vi "Single Calculation.vi"(1 "Array Input":dbl[](array[numeric])) -> (0 "Array Output":dbl[](array[numeric]))   [LabVIEW 2020]
panel:
  out "Charging Voltage":dbl
  out "Total\nTemperature Change":dbl
  out "Energy Loss":dbl
  out "Power Loss":dbl
  out "Charging Time":dbl
  out "Charing Current":dbl
  out "J in 1 NS pair with gap":dbl
  out "Energy (wh/m3) / 1 NS pari with gap":dbl
  out "Energy Density  WH/m3":dbl
  out "Energy Density  WH/Lit":dbl
  out "1 NS Pair Energy / Volume":dbl
  out "1 NS Pair Energy / mass":dbl
  out "Chip Energy Wh":dbl
  out "WH/Lit":dbl
  out "WH/m3":dbl
  out "WH/Kg":dbl
  out "Chip Energy / Volume":dbl
  out "Chip Energy /Mass":dbl
  out "Mass of a Chip":dbl
  out "Volume of a Chip":dbl
  out "Mass NS Pair with Gap":dbl
  out "Volume NS Pair With Gap":dbl
  out "Volume Gap":dbl
  out "Mass Gap":dbl
  out "Delta Temp Change \nDielectric Gap":dbl
  out "Dielectric Thickness  \nGap":dbl
  out "Mass Dielectric \nGap":dbl
  out "Volume Dielectric \nGap":dbl
  out "Delta Temp Change\n SiO2 Gap":dbl
  out "Mass SiO2 Gap":dbl
  out "Sio2 Thickness Gap":dbl
  out "Volume SiO2 Gap":dbl
  out "Volume Si Gap":dbl
  out "Silicon Thickness Gap":dbl
  out "Mass Si Gap":dbl
  out "Delta Temp Change\n Si Gap":dbl
  out "Area B/W NS":dbl
  out "Vol 2 NS":dbl
  out "Mass 2 NS":dbl
  out "Mass 1 NS":dbl
  out "Volume 1 NS":dbl
  out "SiO2 Specfic Heat Capacity 2":dbl
  out "SilO2 Density 2":dbl
  out "Delta Temp Change SiO2 2":dbl
  out "Mass SiO2 2":dbl
  out "Volume SiO2 2":dbl
  out "Dielectric Specfic Heat Capacity":dbl
  out "Dielectric Density":dbl
  out "CNT Specfic Heat Capacity":dbl
  out "CNT Density":dbl
  out "Fe Specfic Heat Capacity":dbl
  out "Fe Density":dbl
  out "Al Specfic Heat Capacity":dbl
  out "Al Density":dbl
  out "Al2O3 Specfic Heat Capacity":dbl
  out "Al2O3 Density":dbl
  out "M1 Specfic Heat Capacity":dbl
  out "M1 Density":dbl
  out "SiO2 Specfic Heat Capacity":dbl
  out "SilO2 Density":dbl
  out "um in 1 inch":dbl
  out "Microns":dbl
  out "Inches":dbl
  out "Energy (Heat; I^2R)":dbl
  out "Delta Temp Change \nDielectric":dbl
  out "Mass Dielectric":dbl
  out "Volume Dielectric":dbl
  out "Delta Temp Change CNT":dbl
  out "Mass CNTs":dbl
  out "Volume CNT":dbl
  out "Delta Temp Change Fe":dbl
  out "Mass Fe":dbl
  out "Volume Fe":dbl
  out "Delta Temp Change Al":dbl
  out "Mass  Al":dbl
  out "Volume Al":dbl
  out "Delta Temp Change Al2O3":dbl
  out "Mass Al2O3":dbl
  out "Volume Al2O3":dbl
  out "Delta Temp Change M1":dbl
  out "Mass M1":dbl
  out "Volume M1":dbl
  out "Delta Temp Change SiO2":dbl
  out "Mass SiO2":dbl
  out "Volume SiO2":dbl
  out "Dielectric Thickness":dbl
  out "CNT Thickness":dbl
  out "Fe Thickness":dbl
  out "Al Thickness":dbl
  out "Al2O3 Thickness":dbl
  out "M1 Thickness":dbl
  out "SiO2 Thickness 2":dbl
  out "Sio2 Thickness":dbl
  out "Silicon Thickness":dbl
  out "m-nm Dielectric":dbl
  out "Dielectric Thickness":dbl
  out "m-nm CNT":dbl
  out "CNT Thickness (CNT Length)":dbl
  out "m-nm Fe":dbl
  out "Fe Thickness":dbl
  out "m-nm Al":dbl
  out "Aluminum Thickness":dbl
  out "Heat Generated (Energy) by Current in Metal films":dbl
  out "Delta Temp Change Si":dbl
  out "Silicon Specfic Heat Capacity":dbl
  out "Silicon Density":dbl
  out "Mass Si":dbl
  out "Volume Si":dbl
  out "m-nm SiO2 2":dbl
  out "Silicon DiOxide Thickness  2":dbl
  out "m-nm Al2O3":dbl
  out "m-nm M1":dbl
  out "Alumina Thickness":dbl
  out "Metal 1 (Ti)":dbl
  out "m-nm SiO2":dbl
  out "m-nm Si":dbl
  out "Silicon DiOxide Thickness":dbl
  out "Silicon Thickness":dbl
  out "Rf for Max i;  R+ C (EDL+Funct)":dbl
  out "Rf for Max i;  R+ C (EDL+Funct+ Analyte)":dbl
  out "Max V_out":dbl
  out "Delta i":dbl
  out "Max i;  R+ C (EDL+Funct+ Analyte)":dbl format="%#_9e"
  out "Max i;  R+ C (EDL+Funct)":dbl format="%#_9e"
  out "V_Zeta":dbl
  out "|Z| of R+ C (EDL+Funct+Analyte)":dbl
  out "|Z| of R+ C (EDL+Funct)":dbl
  out "Delta Total Impedance":dbl
  out "Total Impedance Rs+C(EDS+Funct+Analyte)":dbl
  out "Total Impedance Rs+C(EDS+Funct)":dbl
  out "Series Resistance of Solution":dbl
  out "Freq Hz-MHz":dbl
  out "Impedance of EDL & Functionalization & Analyte":dbl
  out "Impedance of EDL & Functionalization":dbl
  out "Frequency":dbl
  out "Delta C":dbl
  out "Capacitance of ELD & Functionalization & Analyte":dbl
  out "Capacitance of ELD & Functionalization":dbl
  out "C_EDL/ 1 NS":dbl
  out "C_EDL/ 1 CNT":dbl
  out "C EDL by d with Cosh Factor":dbl format="%#_6e"
  out "C EDL by d":dbl
  out "d; EDL Length":dbl
  out "R=kN_a":dbl
  out "F=eN_a":dbl
  out "N_a; Avagadro no":dbl=1.38064852e-23
  out "V  nV-m V-V":dbl
  out "C_EDL/ A":dbl format="%#_6e"
  out "c; Charge on e":dbl=1.6021766208e-19
  out "V zeta":dbl
  out "C in M":dbl
  out "Co nM-M":dbl
  out "T":dbl
  out "k; Boltzmann Constant":dbl=1.38064852e-23
  out "Co; miliMolar (moles/m3)":dbl
  out "er":dbl
  out "eo; Permitivity of Free Space":dbl=8.85418782e-12
  out "z":dbl
  out "Length of CNTs  2":dbl
  out "Dielectric of Molecule 2 Analyte":dbl
  out "Capacitance Functinal Analyte  per unit area":dbl
  out "Capaciatance per CNT Analyte":dbl
  out "Capacitance Functional Analyte per NS":dbl
  out "Capacitance Functional Analyte per NS 2":dbl
  out "Gap B/w NS":dbl
  out "Chip Impedance":dbl
  out "Chip Capacitance":dbl
  out "Chip Energy":dbl
  out "Chip Power":dbl
  out "Freq Hz K; M Hz":dbl
  out "Power":dbl
  out "Frequency":dbl
  out "Impedance":dbl
  out "Voltage":dbl
  out "Energy":dbl
  out "Capacitance of 1 Pair NS":dbl(graph)
  out "Capacitance of 1 Pair NS":dbl
  out "er":dbl
  out "Capacitance Functional Molecules per NS 2":dbl
  out "Capacitance Functional Molecules per NS":dbl
  out "Capaciatance per CNT Functional":dbl
  out "Capacitance Functinal Molecule  per unit area":dbl
  out "Dielectric of Molecule":dbl
  out "Concentration,  M":dbl[unit]
  out "Concentration on 1 NS (Moles/m3)":dbl[unit]
  out "Total Functionalized Molecules on NS":dbl
  out "No of Molecules on 1 CNT Functionalized":dbl
  out "Molecule Length Analyte":dbl
  out "Molecle Area with Gap Analyte":dbl
  out "Volume of Molecule Analyte":dbl
  out "Area of Molecule on CNT surface Analyte":dbl
  out "m-nm Gap Molecules Analyte":dbl caption="m-nm Gap"
  out "Gap Between Molecules Analyte":dbl caption="Gap Between CNTs"
  out "m-nm l Molecule Analyte":dbl
  out "m-nm r Molecule Analyte":dbl caption="m-nm r"
  out "Length of Molecule Analyte":dbl caption="Length of CNTs"
  out "Radius of Molecule Analyte":dbl caption="Radius of CNTs"
  out "Molecule Length":dbl
  out "Molecle Area with Gap":dbl
  out "Volume of Molecule":dbl
  out "Area of Molecule on CNT surface":dbl
  out "m-nm Gap Molecules":dbl caption="m-nm Gap"
  out "Gap Between Molecules":dbl caption="Gap Between CNTs"
  out "m-nm l Molecule":dbl
  out "m-nm r Molecule":dbl caption="m-nm r"
  out "Length of Molecule":dbl caption="Length of CNTs"
  out "Radius of Molecule":dbl caption="Radius of CNTs"
  out "NS Width":dbl
  out "No of NS Pairs on Chip":dbl
  out "Gap n-m":dbl
  out "Gap B/W NS":dbl
  out "m-nm LChip":dbl
  out "m-nm WChip":dbl
  out "Length of Chip":dbl
  out "Width of Chip":dbl
  out "Surface Area 1 NS":dbl
  out "# of CNTs in 1 NS":dbl format="%#_6e"
  out "Area 1 CNT & Gap":dbl
  out "NS Length":dbl
  out "NS Base Area":dbl
  out "CNT Radius":dbl
  out "CNT Base Area":dbl
  out "XY Graph":cluster{"X":dbl[], "Y":dbl[]}[](graph)
  out "m-nm NS Base":dbl caption="m-nm 4"
  out "m-nm WB":dbl
  out "Length of Base":dbl
  out "Width of Base":dbl
  out "m-nm Gap":dbl
  out "Gap Between CNTs":dbl
  out "Surface Area of 1 CNT":dbl
  out "m-nm l":dbl
  out "m-nm r":dbl
  out "Length of CNTs":dbl
  out "Radius of CNTs":dbl
  # "CAP"
  # "Chip CAP"
  # "Chip NanoStructure"
  # "CNT Nanostructure"
  # "CAP Design"
  # "Nano Structure Material Stack"
  # "Constants for Materials in Stack"
  # "Nano Structure"
  # "Charging/Discharging"
  # "Chip"
  # "Dielectric =1/2 of Gap B/w NS"
  # "Analyte Molecule"
  # "Functionalization Molecule"
  # "Analyte Attached to Functionalized  NanoStructure"
  # "TiO2: 4260 kg/m3\nHafnium Odide: 9680"
  # "GAP B/W NS  Material"
  # "Capacitance of Analyte Molecule on NanoStructure"
  # "Functionalized NanoStructure"
  # "Mass and Volume of NS Pair"
  # "Molecule Fnctionalization"
  # "Capacitance of Functional Molecule on NanoStructure"
  # "Mass and Volume of Chip"
  # "Echem & Electrical Signals"
  # "Electric Double Layer; EDL"
  # "Constants"
  # "Cosh(zeV_zeta/2kT)"
  # "Potentiostat"
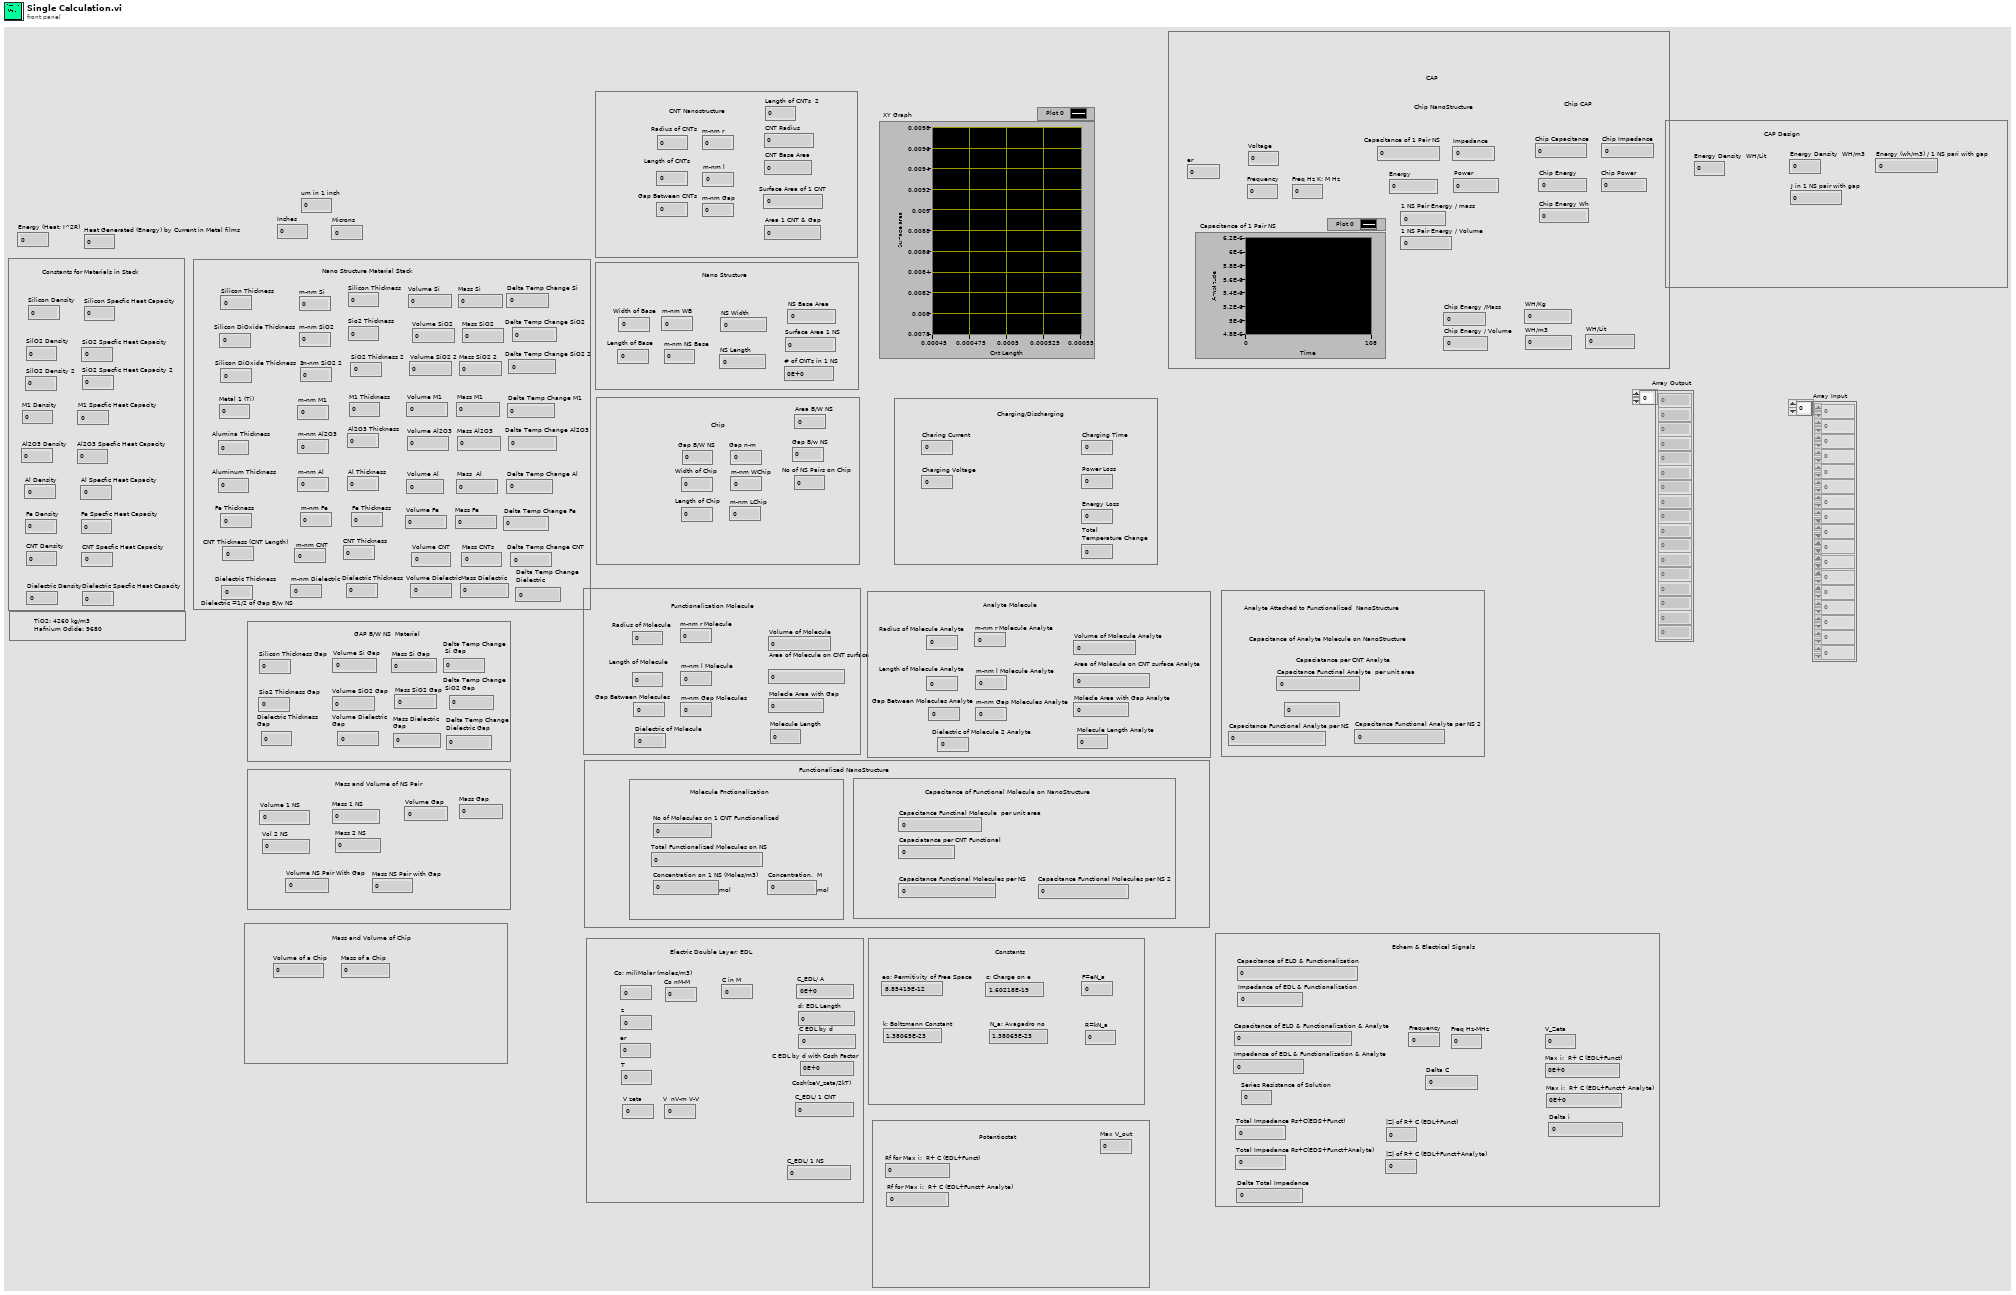
[diagram p1: front panel]
types:
  T1 = cluster{"Array Input[0]":dbl, "Array Input[1]":dbl, "Array Input[2]":dbl, "Array Input[3]":dbl, "Array Input[4]":dbl, "Array Input[5]":dbl, "Array Input[6]":dbl, "Array Input[7]":dbl, "Array Input[8]":dbl, "Array Input[9]":dbl, "Array Input[10]":dbl, "Array Input[11]":dbl, "Array Input[12]":dbl, "Array Input[13]":dbl, "Array Input[14]":dbl, "Array Input[15]":dbl, "Array Input[16]":dbl, "Array Input[17]":dbl, "Array Input[18]":dbl, "Array Input[19]":dbl, "Array Input[20]":dbl, "Array Input[21]":dbl, "Array Input[22]":dbl, "Array Input[23]":dbl, "Array Input[24]":dbl, "Array Input[25]":dbl, "Array Input[26]":dbl, "Array Input[27]":dbl, "Array Input[28]":dbl, "Array Input[29]":dbl, "Array Input[30]":dbl, "Array Input[31]":dbl, "Array Input[32]":dbl, "Array Input[33]":dbl, "Array Input[34]":dbl, "Array Input[35]":dbl, "Array Input[36]":dbl, "Array Input[37]":dbl, "Array Input[38]":dbl, "Array Input[39]":dbl, "Array Input[40]":dbl, "Array Input[41]":dbl, "Array Input[42]":dbl, "Array Input[43]":dbl, "Array Input[44]":dbl, "Array Input[45]":dbl, "Array Input[46]":dbl, "Array Input[47]":dbl, "Array Input[48]":dbl, "Array Input[49]":dbl, "Array Input[50]":dbl, "Array Input[51]":dbl, "Array Input[52]":dbl, "Array Input[53]":dbl, "Array Input[54]":dbl, "Array Input[55]":dbl, "Array Input[56]":dbl, "Array Input[57]":dbl, "Array Input[58]":dbl, "Array Input[59]":dbl, "Array Input[60]":dbl, "Array Input[61]":dbl, "Array Input[62]":dbl, "Array Input[63]":dbl}
  T2 = cluster{"Capacitance of 1 Pair NS":dbl, "Energy":dbl, dbl, dbl, "Impedance":dbl, "Power":dbl, dbl, dbl, "Chip Capacitance":dbl, "Chip Energy":dbl, dbl, dbl, dbl, "Chip Impedance":dbl, "Chip Power":dbl, dbl, dbl, dbl, dbl, "Volume of Molecule":dbl, "Area of Molecule on CNT surface":dbl, "Molecle Area with Gap":dbl, "Molecule Length":dbl, "Capacitance Functinal Analyte  per unit area":dbl, "Capaciatance per CNT":dbl, "Capacitance Functional Analyte per NS 2":dbl, "Capacitance Functional Analyte per NS 2":dbl, "Volume of Molecule":dbl, "Area of Molecule on CNT surface":dbl, "Molecle Area with Gap":dbl, "Molecule Length":dbl, "No of Molecules on 1 CNT Functionalized ":dbl, "Total Functionalized Molecules on NS":dbl, dbl, dbl, "Capacitance Functinal Molecule  per unit area":dbl, "Capaciatance per CNT":dbl, "Capacitance Functional Molecules per NS":dbl, "Capacitance Functional Molecules per NS 2":dbl, "eo; Permitivity of Free Space":dbl, "c; Charge on e":dbl, "F=eN_a":dbl, "k; Boltzmann Constant":dbl, "N_a; Avagadro no":dbl, "R=kN_a":dbl, "C in M":dbl, "C_EDL/ A":dbl, "d; EDL Length":dbl, "C EDL by d":dbl, "C EDL by d with Cosh Factor":dbl, "C_EDL/ 1 CNT":dbl, "C_EDL/ 1 NS":dbl, dbl, dbl, "Capacitance of ELD & Functionalization":dbl, "Impedance of EDL & Functionalization":dbl, "Capacitance of ELD & Functionalization & Analyte":dbl, "Impedance of EDL & Functionalization & Analyte":dbl, "Total Impedance Rs+C(EDS+Funct)":dbl, "Total Impedance Rs+C(EDS+Funct+Analyte)":dbl, "Delta Total Impedance":dbl, "Delta C":dbl, "|Z| of R+ C (EDL+Funct)":dbl, "|Z| of R+ C (EDL+Funct+Analyte)":dbl, "V_Zeta out":dbl, "Max i;  R+ C (EDL+Funct) ":dbl, "Max i;  R+ C (EDL+Funct+ Analyte) ":dbl, "Delta i":dbl, dbl, dbl, dbl, dbl, dbl, dbl, dbl, dbl, dbl, dbl, "Silicon Thickness out":dbl, "Sio2 Thickness":dbl, "Dielectric Thickness  out":dbl, "Volume Si":dbl, "Volume SiO2":dbl, "Volume Dielectric":dbl, "Mass Si":dbl, "Mass SiO2":dbl, "Mass Dielectric":dbl, "Delta Temp Change Si":dbl, "Delta Temp Change SiO2":dbl, "Delta Temp Change \nDielectric":dbl, "Array Input[1]":dbl, dbl, "Array Input[4]":dbl, "Array Input[29]":dbl, "Silicon Thickness out":dbl, "Sio2 Thickness":dbl, "SiO2 Thickness 2":dbl, "M1 Thickness":dbl, "Al2O3 Thickness":dbl, "Al Thickness":dbl, "Fe Thickness 2":dbl, "CNT Thickness":dbl, "Dielectric Thickness  out":dbl, "Volume Si":dbl, "Volume SiO2":dbl, "Volume SiO2 2":dbl, "Volume M1":dbl, "Volume Al2O3":dbl, "Volume Al":dbl, "Volume Fe":dbl, "Volume CNT":dbl, "Volume Dielectric":dbl, "Mass Si":dbl, "Mass SiO2":dbl, "Mass SiO2 2":dbl, "Mass M1":dbl, "Mass Al2O3":dbl, "Mass  Al":dbl, "Mass Fe":dbl, "Mass CNTs":dbl, "Mass Dielectric":dbl, "Delta Temp Change Si":dbl, "Delta Temp Change SiO2":dbl, "Delta Temp Change SiO2 2":dbl, "Delta Temp Change M1":dbl, "Delta Temp Change Al2O3":dbl, "Delta Temp Change Al":dbl, "Delta Temp Change Fe":dbl, "Delta Temp Change CNT":dbl, "Delta Temp Change \nDielectric":dbl, dbl, "y":dbl, dbl, dbl, "Gap B/w NS":dbl, "No of NS Pairs on Chip":dbl, "NS Width":dbl, "NS Length":dbl, "NS Base Area":dbl, "Surface Area 1 NS":dbl, "# of CNTs in 1 NS":dbl, "Length of CNTs ":dbl, "CNT Radius":dbl, "CNT Base Area":dbl, "Surface Area of 1 CNT":dbl, "Area 1 CNT & Gap":dbl, "Silicon Density":dbl, "SilO2 Density":dbl, "SilO2 Density 2":dbl, "M1 Density":dbl, "Al2O3 Density":dbl, "Al Density":dbl, "Fe Density":dbl, "CNT Density":dbl, "Dielectric Density":dbl, "Silicon Specfic Heat Capacity":dbl, "SiO2 Specfic Heat Capacity":dbl, "SiO2 Specfic Heat Capacity 2":dbl, "M1 Specfic Heat Capacity":dbl, "Al2O3 Specfic Heat Capacity":dbl, "Al Specfic Heat Capacity":dbl, "Fe Specfic Heat Capacity":dbl, "CNT Specfic Heat Capacity":dbl, "Dielectric Specfic Heat Capacity":dbl, dbl, dbl, dbl, dbl}
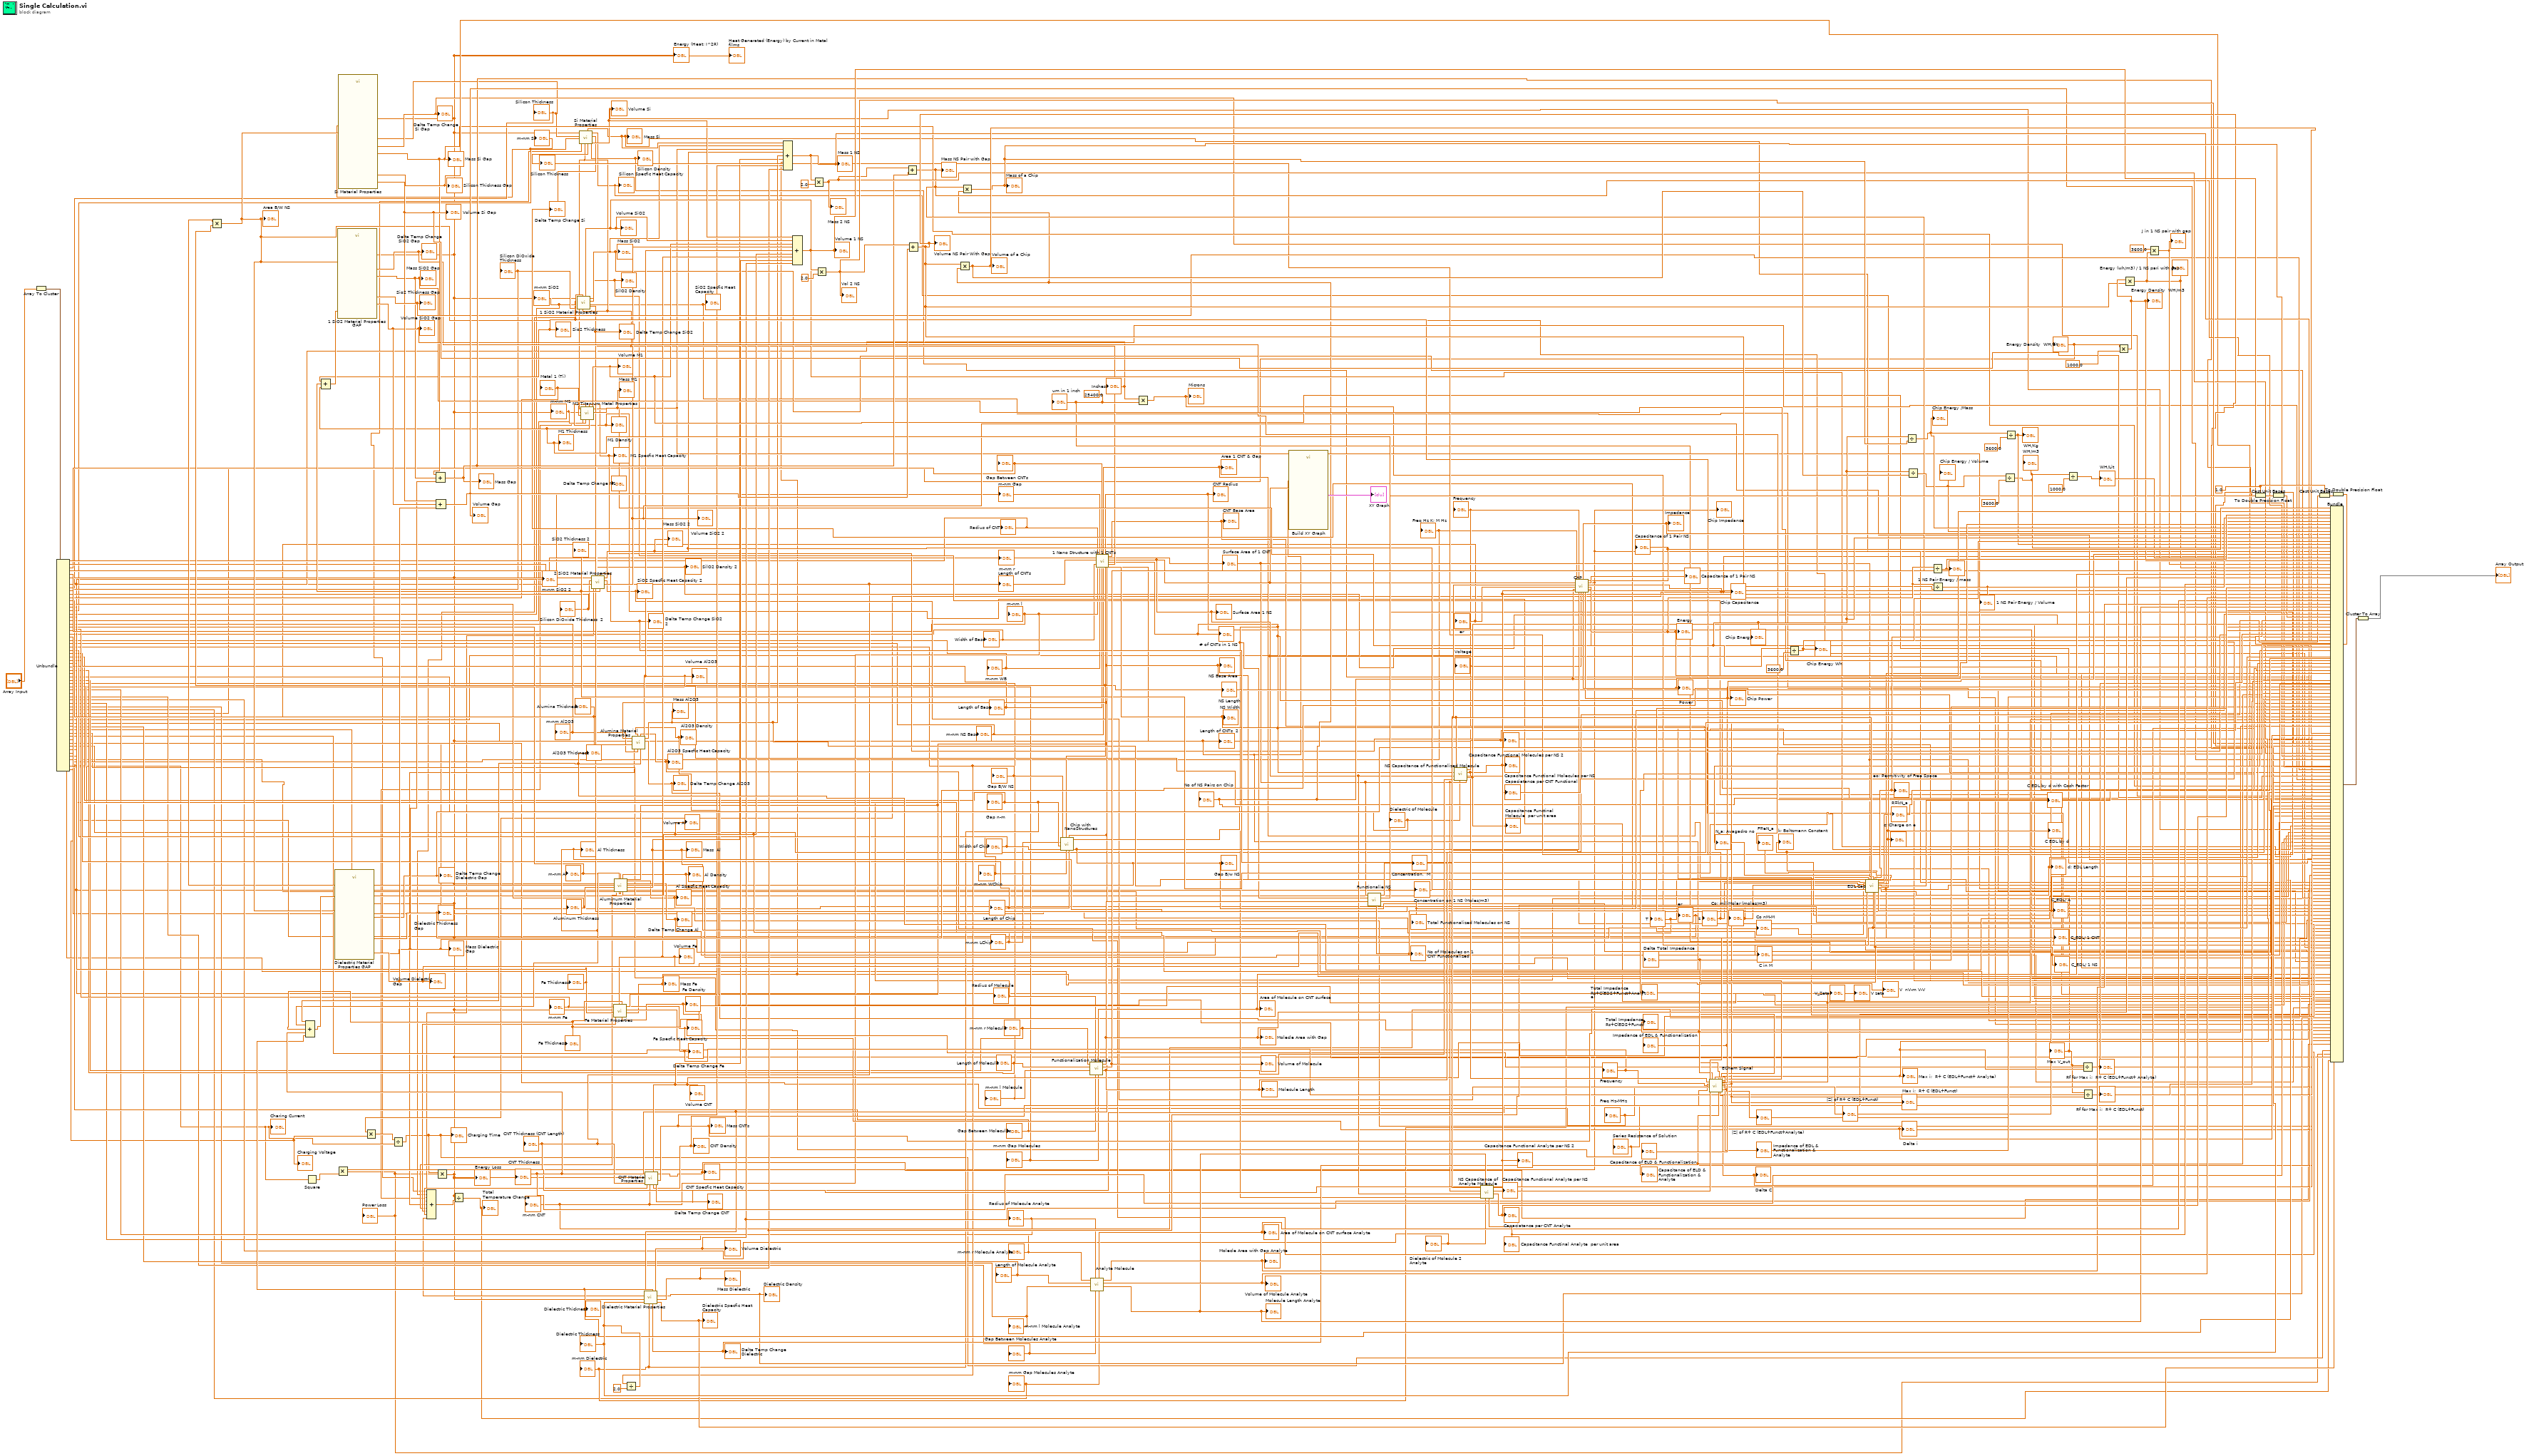
[diagram p0: block diagram]
diagram:
  w205 = 1.0
  w116 = 25400.0 ("y")
  n1 = Array To Cluster(array="Array Input") -> (cluster=w246:T1)
  n2 = Unbundle(w246) -> ("Array Input[0]"=w82:dbl, "Array Input[1]"=w81:dbl, "Array Input[2]"=w80:dbl, "Array Input[3]"=w79:dbl, "Array Input[4]"=w78:dbl, "Array Input[5]"=w77:dbl, "Array Input[7]"=w76:dbl, "Array Input[8]"=w75:dbl, "Array Input[9]"=w74:dbl, "Array Input[10]"=w73:dbl, "Array Input[11]"=w72:dbl, "Array Input[12]"=w71:dbl, "Array Input[13]"=w70:dbl, "Array Input[14]"=w69:dbl, "Array Input[15]"=w68:dbl, "Array Input[16]"=w67:dbl, "Array Input[17]"=w66:dbl, "Array Input[18]"=w65:dbl, "Array Input[19]"=w64:dbl, "Array Input[20]"=w63:dbl, "Array Input[21]"=w62:dbl, "Array Input[22]"=w61:dbl, "Array Input[23]"=w60:dbl, "Array Input[24]"=w59:dbl, "Array Input[25]"=w58:dbl, "Array Input[26]"=w57:dbl, "Array Input[27]"=w56:dbl, "Array Input[28]"=w55:dbl, "Array Input[29]"=w54:dbl, "Array Input[30]"=w53:dbl, "Array Input[31]"=w52:dbl, "Array Input[32]"=w51:dbl, "Array Input[33]"=w50:dbl, "Array Input[34]"=w49:dbl, "Array Input[35]"=w48:dbl, "Array Input[36]"=w47:dbl, "Array Input[37]"=w46:dbl, "Array Input[38]"=w45:dbl, "Array Input[39]"=w44:dbl, "Array Input[40]"=w43:dbl, "Array Input[41]"=w42:dbl, "Array Input[42]"=w41:dbl, "Array Input[43]"=w40:dbl, "Array Input[44]"=w39:dbl, "Array Input[45]"=w38:dbl, "Array Input[46]"=w37:dbl, "Array Input[47]"=w36:dbl, "Array Input[48]"=w35:dbl, "Array Input[49]"=w34:dbl, "Array Input[50]"=w33:dbl, "Array Input[51]"=w32:dbl, "Array Input[52]"=w31:dbl, "Array Input[53]"=w30:dbl, "Array Input[54]"=w29:dbl, "Array Input[55]"=w28:dbl, "Array Input[56]"=w27:dbl, "Array Input[57]"=w26:dbl, "Array Input[58]"=w25:dbl, "Array Input[59]"=w24:dbl, "Array Input[60]"=w23:dbl, "Array Input[61]"=→"V  nV-m V-V":dbl, "Array Input[62]"=w17:dbl, "Array Input[63]"=w19:dbl)  [unwired: 1 out]
  "Radius of CNTs" <- w82
  "Length of CNTs" <- w81
  "m-nm r" <- w79
  "m-nm l" <- w78
  "Gap Between CNTs" <- w80
  "m-nm Gap" <- w77
  "Width of Base" <- w61
  "Length of Base" <- w60
  "m-nm WB" <- w59
  "m-nm NS Base" <- w58
  "Width of Chip" <- w56
  "Length of Chip" <- w55
  "m-nm WChip" <- w53
  "m-nm LChip" <- w52
  "Gap B/W NS" <- w57
  "Gap n-m" <- w54
  "Radius of Molecule" <- w51
  "Length of Molecule" <- w50
  "m-nm r Molecule" <- w47
  "m-nm l Molecule" <- w46
  "Gap Between Molecules" <- w49
  "m-nm Gap Molecules" <- w45
  "Radius of Molecule Analyte" <- w44
  "Length of Molecule Analyte" <- w43
  "m-nm r Molecule Analyte" <- w40
  "m-nm l Molecule Analyte" <- w39
  "Gap Between Molecules Analyte" <- w42
  "m-nm Gap Molecules Analyte" <- w38
  "Dielectric of Molecule" <- w48
  "er" <- w36
  "Voltage" <- w35
  "Frequency" <- w34
  "Freq Hz K; M Hz" <- w33
  "Dielectric of Molecule 2 Analyte" <- w41
  "z" <- w27
  "er" <- w26
  "Co; miliMolar (moles/m3)" <- w28
  "T" <- w25
  "Co nM-M" <- w23
  "V zeta" <- w24
  "Frequency" <- w30
  "Freq Hz-MHz" <- w29
  "Series Resistance of Solution" <- w31
  "Max V_out" <- w32
  "Silicon Thickness" <- w75
  "Silicon DiOxide Thickness" <- w74
  "m-nm Si" <- w68
  "m-nm SiO2" <- w67
  "Metal 1 (Ti)" <- w72
  "Alumina Thickness" <- w71
  "m-nm M1" <- w65
  "m-nm Al2O3" <- w64
  "Silicon DiOxide Thickness  2" <- w73
  "m-nm SiO2 2" <- w66
  "Aluminum Thickness" <- w70
  "m-nm Al" <- w63
  "Fe Thickness" <- w69
  "m-nm Fe" <- w62
  "CNT Thickness (CNT Length)" <- w81
  "m-nm CNT" <- w78
  "m-nm Dielectric" <- w54
  "Inches" <- w76
  "Energy Density  WH/Lit" <- w37
  "Charing Current" <- w17
  "Charging Voltage" <- w19
  n3 = Square(x=w17) -> (x^2=w16:dbl)
  n4 = Divide(x=w57, y=2.0) -> (x/y=w152:dbl)
  "Dielectric Thickness" <- w152
  n5 = call "Functionalization Molecule.vi"("m-nm Gap Molecules"=w45, "Gap Between Molecules"=w49, "Radius of Molecule"=w51, "m-nm l Molecule"=w46, "Length of Molecule"=w50, "m-nm r Molecule"=w47) -> ("Molecule Length"=w225:dbl, "Volume of Molecule"=w228:dbl, "Molecle Area with Gap"=w226:dbl, "Area of Molecule on CNT surface"=w227:dbl)  [unwired: 2 in]
  "Area of Molecule on CNT surface" <- w227
  "Volume of Molecule" <- w228
  "Molecle Area with Gap" <- w226
  "Molecule Length" <- w225
  n6 = call "Analyte Molecule.vi"("m-nm Gap Molecules"=w38, "Gap Between Molecules"=w42, "Radius of Molecule"=w44, "m-nm l Molecule"=w39, "Length of Molecule"=w43, "m-nm r Molecule"=w40) -> ("Molecule Length"=w218:dbl, "Volume of Molecule"=w221:dbl, "Molecle Area with Gap"=w219:dbl, "Area of Molecule on CNT surface"=w220:dbl)  [unwired: 2 in]
  "Area of Molecule on CNT surface Analyte" <- w220
  "Volume of Molecule Analyte" <- w221
  "Molecle Area with Gap Analyte" <- w219
  "Molecule Length Analyte" <- w218
  n7 = call "1 Nano Structure with 1 CNTs.vi"("Radius of CNTs"=w82, "m-nm r"=w79, "Length of CNTs"=w81, "m-nm l"=w78, "Width of Base"=w61, "m-nm Gap"=w77, "m-nm WB"=w59, "Gap Between CNTs"=w80, "Length of Base"=w60, "m-nm NS Base"=w58) -> ("Length of CNTs"=w106:dbl, "Area 1 CNT & Gap"=w102:dbl, "CNT Radius"=w105:dbl, "NS Length"=w110:dbl, "CNT Base Area"=w104:dbl, "Surface Area of 1 CNT"=w103:dbl, "Surface Area 1 NS"=w108:dbl, "# of CNTs in 1 NS"=w107:dbl, "NS Base Area"=w109:dbl, "NS Width"=w111:dbl)
  "Surface Area of 1 CNT" <- w103
  "CNT Base Area" <- w104
  "CNT Radius" <- w105
  "NS Base Area" <- w109
  "NS Length" <- w110
  "Area 1 CNT & Gap" <- w102
  "# of CNTs in 1 NS" <- w107
  "Surface Area 1 NS" <- w108
  "NS Width" <- w111
  "Length of CNTs  2" <- w106
  n8 = call "Chip with NanoStructures.vi"("Length of Chip"=w55, "NS Base Area"=w109, "m-nm WChip"=w53, "NS Length"=w110, "Width of Chip"=w56, "Gap n-m"=w54, "m-nm LChip"=w52, "Gap B/W NS"=w57) -> ("Gap B/w NS"=w113:dbl, "No of NS Pairs on Chip"=w112:dbl)  [unwired: 2 in]
  "No of NS Pairs on Chip" <- w112
  "Gap B/w NS" <- w113
  n9 = Multiply(x=w113, y=w110) -> (x*y=w114:dbl)
  "Area B/W NS" <- w114
  n10 = Multiply(x=w76, y=w116) -> (x*y=w115:dbl)
  "Microns" <- w115
  n11 = call "Build XY Graph"("Y Input"=w108, "X Input"=w106) -> ("XY Graph"=→"XY Graph":cluster{"X":dbl[], "Y":dbl[]}[])  [unwired: 8 in, 1 out]
  n12 = call "Functionalie NS.vi"("Molecle Area with Gap"=w226, "# of CNTs in 1 NS"=w107, "Surface Area of 1 CNT"=w103) -> ("Total Functionalized Molecules on NS"=w216:dbl, "Concentration on 1 NS (Moles/m3)"=w210:ext[unit], "Concentration,  M"=w207:ext[unit], "No of Molecules on 1 CNT Functionalized"=w217:dbl)  [unwired: 5 in]
  "No of Molecules on 1 CNT Functionalized" <- w217
  "Total Functionalized Molecules on NS" <- w216
  "Concentration on 1 NS (Moles/m3)" <- w210
  "Concentration,  M" <- w207
  n13 = call "EDL Cap.vi"("T"=w25, "er"=w26, "z"=w27, "Co; miliMolar (moles/m3)"=w28, "Co nM-M"=w23, "V zeta"=w24, "# of CNTs in 1 NS"=w107, "Surface Area of 1 CNT"=w103) -> ("V_Zeta"=w259:dbl, "eo; Permitivity of Free Space 2"=w261:dbl, "N_a; Avagadro no"=w199:dbl, "C in M"=w197:dbl, "eo; Permitivity of Free Space"=w203:dbl, "C_EDL/ 1 NS"=w191:dbl, "k; Boltzmann Constant"=w200:dbl, "C_EDL/ 1 CNT"=w192:dbl, "F=eN_a"=w201:dbl, "R=kN_a"=w198:dbl, "c; Charge on e"=w202:dbl, "C EDL by d with Cosh Factor"=w193:dbl, "C EDL by d"=w194:dbl, "d; EDL Length"=w195:dbl, "C_EDL/ A"=w196:dbl)  [unwired: 5 in]
  "eo; Permitivity of Free Space" <- w203
  "k; Boltzmann Constant" <- w200
  "C in M" <- w197
  "c; Charge on e" <- w202
  "C_EDL/ A" <- w196
  "N_a; Avagadro no" <- w199
  "F=eN_a" <- w201
  "R=kN_a" <- w198
  "d; EDL Length" <- w195
  "C EDL by d" <- w194
  "C EDL by d with Cosh Factor" <- w193
  "C_EDL/ 1 CNT" <- w192
  "C_EDL/ 1 NS" <- w191
  n14 = call "NS Capacitance of Functionalized Molecule.vi"("SA of 1 CNT"=w103, "Dielectric of Molecule"=w48, "Molecule Length"=w225, "Surface Area 1 NS"=w108, "# of CNTs"=w107, "Permitivity of Free Space"=w261) -> ("Capaciatance per CNT"=w214:dbl, "Capacitance Functional Molecules per NS"=w213:dbl, "Capacitance Functional Molecules per NS 2"=w212:dbl, "Capacitance Functinal Molecule  per unit area"=w215:dbl)  [unwired: 2 in]
  "Capacitance Functinal Molecule  per unit area" <- w215
  "Capaciatance per CNT Functional" <- w214
  "Capacitance Functional Molecules per NS" <- w213
  "Capacitance Functional Molecules per NS 2" <- w212
  n15 = call "NS Capacitance of Analyte Molecule.vi"("Dielectric of Molecule Analyte"=w41, "Molecule Length"=w218, "# of CNTs"=w107, "Surface Area 1 NS"=w108, "Surface Area of 1 CNT"=w103, "Permitivity of Free Space"=w261) -> ("Capaciatance per CNT"=w223:dbl, "Capacitance Functional Analyte per NS"=w260:dbl, "Capacitance Functional Analyte per NS 2"=w222:dbl, "Capacitance Functinal Analyte  per unit area"=w224:dbl)  [unwired: 2 in]
  "Capacitance Functional Analyte per NS 2" <- w222
  "Capacitance Functional Analyte per NS" <- w260
  "Capaciatance per CNT Analyte" <- w223
  "Capacitance Functinal Analyte  per unit area" <- w224
  n16 = call "CAP.vi"("Freq Hz K; M Hz"=w33, "Surface Area 1 NS"=w108, "Permitivity of Free Space"=w261, "er"=w36, "No of NS Pairs on Chip"=w112, "Frequency"=w34, "Gap B/w NS"=w113, "Voltage"=w35) -> ("Impedance"=w241:dbl, "Power"=w240:dbl, "Chip Impedance"=w15:dbl, "Chip Power"=w233:dbl, "Capacitance of 1 Pair NS"=w245:dbl, "Capacitance of 1 Pair"=→"Capacitance of 1 Pair NS":dbl, "Chip Capacitance"=w20:dbl, "Chip Energy"=w237:dbl, "Energy"=w244:dbl)  [unwired: 3 in]
  "Capacitance of 1 Pair NS" <- w245
  "Energy" <- w244
  "Impedance" <- w241
  "Power" <- w240
  "Chip Power" <- w233
  "Chip Energy" <- w237
  "Chip Capacitance" <- w20
  "Chip Impedance" <- w15
  n17 = Multiply(x=w15, y=w16) -> (x*y=w1:dbl)
  "Power Loss" <- w1
  n18 = Multiply(x=w20, y=w19) -> (x*y=w18:dbl)
  n19 = Divide(x=w18, y=w17) -> (x/y=w2:dbl)
  "Charging Time" <- w2
  n20 = Multiply(x=w2, y=w1) -> (x*y=w4:dbl)
  "Heat Generated (Energy) by Current in Metal films" <- w4
  "Energy (Heat; I^2R)" <- w4
  "Energy Loss" <- w4
  n21 = call "Si Material Properties.vi"("NS Base Area"=w114, "m-nm Si"=w68, "Silicon Thickness in"=w75, "Energy (Heat; I^2R)"=w4) -> ("Volume Si"=w161:dbl, "Delta Temp Change Si"=w155:dbl, "Silicon Thickness out"=w164:dbl, "Mass Si"=w158:dbl)  [unwired: 1 in, 3 out]
  "Delta Temp Change\n Si Gap" <- w155
  "Mass Si Gap" <- w158
  "Silicon Thickness Gap" <- w164
  "Volume Si Gap" <- w161
  n22 = call "1 SiO2 Material Properties.vi"("NS Base Area"=w109, "Silicon DiOxide Thickness  in"=w74, "m-nm SiO2 in"=w67, "Energy (Heat; I^2R)"=w4) -> ("SiO2 Specfic Heat Capacity"=w91:dbl, "Mass SiO2"=w132:dbl, "SilO2 Density"=w100:dbl, "Delta Temp Change SiO2"=w124:dbl, "Volume SiO2"=w141:dbl, "Sio2 Thickness"=w142:dbl, "mc"=w6:dbl)  [unwired: 1 in]
  "Sio2 Thickness" <- w142
  "Volume SiO2" <- w141
  "Mass SiO2" <- w132
  "Delta Temp Change SiO2" <- w124
  "SilO2 Density" <- w100
  "SiO2 Specfic Heat Capacity" <- w91
  n23 = call "Si Material Properties.vi"("NS Base Area"=w109, "m-nm Si"=w68, "Silicon Thickness in"=w75, "Energy (Heat; I^2R)"=w4) -> ("Volume Si"=w143:dbl, "Silicon Density"=w101:dbl, "Delta Temp Change Si"=w125:dbl, "Silicon Specfic Heat Capacity"=w92:dbl, "Silicon Thickness out"=w151:dbl, "Mass Si"=w133:dbl, "mc"=w5:dbl)  [unwired: 1 in]
  "Volume Si" <- w143
  "Mass Si" <- w133
  "Silicon Density" <- w101
  "Silicon Specfic Heat Capacity" <- w92
  "Delta Temp Change Si" <- w125
  "Silicon Thickness" <- w151
  n24 = call "M1 Titanium Metal Properties.vi"("m-nm M1"=w65, "Metal 1 (Ti)"=w72, "Energy (Heat; I^2R)"=w4, "NS Base Area"=w109) -> ("Volume M1"=w139:dbl, "Mass M1"=w130:dbl, "Delta Temp Change M1"=w122:dbl, "M1 Thickness"=w149:dbl, "M1 Specfic Heat Capacity"=w89:dbl, "M1 Density"=w98:dbl, "mc"=w7:dbl)  [unwired: 1 in]
  "M1 Thickness" <- w149
  "Volume M1" <- w139
  "Mass M1" <- w130
  "Delta Temp Change M1" <- w122
  "M1 Density" <- w98
  "M1 Specfic Heat Capacity" <- w89
  n25 = call "2 SiO2 Material Properties.vi"("NS Base Area"=w109, "m-nm SiO2 in"=w66, "Silicon DiOxide Thickness  in"=w73, "Energy (Heat; I^2R)"=w4) -> ("Volume SiO2 2"=w140:dbl, "SiO2 Specfic Heat Capacity 2"=w90:dbl, "Mass SiO2 2"=w131:dbl, "SiO2 Thickness 2"=w150:dbl, "Delta Temp Change SiO2 2"=w123:dbl, "SilO2 Density 2"=w99:dbl, "mc"=w8:dbl)  [unwired: 1 in]
  "SiO2 Thickness 2" <- w150
  "Volume SiO2 2" <- w140
  "Mass SiO2 2" <- w131
  "Delta Temp Change SiO2 2" <- w123
  "SilO2 Density 2" <- w99
  "SiO2 Specfic Heat Capacity 2" <- w90
  n26 = Compound Arithmetic op=ADD(w142, w150, w149) -> (w254:dbl)
  n27 = call "1 SiO2 Material Properties GAP.vi"("NS Base Area"=w114, "Sio2 Thickness 2"=w254, "Energy (Heat; I^2R)"=w4) -> ("Mass SiO2"=w157:dbl, "Delta Temp Change SiO2"=w154:dbl, "Volume SiO2"=w160:dbl, "Sio2 Thickness"=w163:dbl)  [unwired: 3 in, 2 out]
  "Volume SiO2 Gap" <- w160
  "Sio2 Thickness Gap" <- w163
  "Mass SiO2 Gap" <- w157
  "Delta Temp Change\n SiO2 Gap" <- w154
  n28 = call "Fe Material Properties.vi"("m-nm Fe"=w62, "Fe Thickness"=w69, "Energy (Heat; I^2R)"=w4, "NS Base Area"=w109) -> ("Mass Fe"=w22:dbl, "Delta Temp Change Fe"=w119:dbl, "Fe Specfic Heat Capacity"=w86:dbl, "Fe Density"=w95:dbl, "Fe Thickness 2"=w146:dbl, "Volume Fe"=w136:dbl, "mc"=w11:dbl)  [unwired: 1 in]
  "Fe Thickness" <- w146
  "Volume Fe" <- w136
  "Mass Fe" <- w22
  "Delta Temp Change Fe" <- w119
  "Fe Density" <- w95
  "Fe Specfic Heat Capacity" <- w86
  n29 = call "Aluminum Material Properties.vi"("m-nm Al"=w63, "Aluminum Thickness"=w70, "Energy (Heat; I^2R)"=w4, "NS Base Area"=w109) -> ("Mass  Al"=w128:dbl, "Delta Temp Change Al"=w120:dbl, "Al Specfic Heat Capacity"=w87:dbl, "Volume Al"=w137:dbl, "Al Density"=w96:dbl, "Al Thickness"=w147:dbl, "mc"=w10:dbl)  [unwired: 1 in]
  "Al Thickness" <- w147
  "Volume Al" <- w137
  "Mass  Al" <- w128
  "Delta Temp Change Al" <- w120
  "Al Density" <- w96
  "Al Specfic Heat Capacity" <- w87
  n30 = call "Alumina Material Properties.vi"("m-nm Al2O3"=w64, "Alumina Thickness"=w71, "Energy (Heat; I^2R)"=w4, "NS Base Area"=w109) -> ("Volume Al2O3"=w138:dbl, "Delta Temp Change Al2O3"=w121:dbl, "Mass Al2O3"=w129:dbl, "Al2O3 Thickness"=w148:dbl, "Al2O3 Specfic Heat Capacity"=w88:dbl, "Al2O3 Density"=w97:dbl, "mc"=w9:dbl)  [unwired: 1 in]
  "Al2O3 Thickness" <- w148
  "Volume Al2O3" <- w138
  "Mass Al2O3" <- w129
  "Delta Temp Change Al2O3" <- w121
  "Al2O3 Density" <- w97
  "Al2O3 Specfic Heat Capacity" <- w88
  n31 = call "Dielectric Material Properties.vi"("m-nm Dielectric"=w54, "Dielectric Thickness  in"=w152, "Energy (Heat; I^2R)"=w4, "NS Base Area"=w109) -> ("Dielectric Specfic Heat Capacity"=w84:dbl, "Mass Dielectric"=w126:dbl, "Dielectric Density"=w93:dbl, "Volume Dielectric"=w134:dbl, "Delta Temp Change \nDielectric"=w117:dbl, "Dielectric Thickness  out"=w144:dbl, "mc"=w13:dbl)  [unwired: 1 in]
  "Dielectric Thickness" <- w144
  "Volume Dielectric" <- w134
  "Mass Dielectric" <- w126
  "Delta Temp Change \nDielectric" <- w117
  "Dielectric Density" <- w93
  "Dielectric Specfic Heat Capacity" <- w84
  n32 = call "CNT Material Properties.vi"("m-nm CNT"=w78, "CNT Thickness (CNT Length)"=w81, "Energy (Heat; I^2R)"=w4, "NS Base Area"=w109) -> ("Mass CNTs"=w127:dbl, "Delta Temp Change CNT"=w118:dbl, "CNT Specfic Heat Capacity"=w85:dbl, "CNT Density"=w94:dbl, "Volume CNT"=w135:dbl, "CNT Thickness"=w145:dbl, "mc"=w12:dbl)  [unwired: 1 in]
  "CNT Thickness" <- w145
  "Volume CNT" <- w135
  "Mass CNTs" <- w127
  "Delta Temp Change CNT" <- w118
  "CNT Density" <- w94
  "CNT Specfic Heat Capacity" <- w85
  n33 = Compound Arithmetic op=ADD(w148, w147, w146, w145, w144) -> (w255:dbl)
  n34 = call "Dielectric Material Properties GAP.vi"("Dielectric Thickness Total"=w255, "Energy (Heat; I^2R)"=w4, "NS Base Area"=w114) -> ("Mass Dielectric"=w156:dbl, "Volume Dielectric"=w159:dbl, "Delta Temp Change \nDielectric"=w153:dbl, "Dielectric Thickness  out"=w162:dbl)  [unwired: 3 in, 2 out]
  "Volume Dielectric \nGap" <- w159
  "Mass Dielectric \nGap" <- w156
  "Dielectric Thickness  \nGap" <- w162
  "Delta Temp Change \nDielectric Gap" <- w153
  n35 = Compound Arithmetic op=ADD(w5, w6, w7, w8, w9, w10, w11, w12, w13) -> (w14:dbl)
  n36 = Compound Arithmetic op=ADD(w158, w157, w156) -> (w165:dbl)
  "Mass Gap" <- w165
  n37 = Compound Arithmetic op=ADD(w161, w160, w159) -> (w166:dbl)
  "Volume Gap" <- w166
  n38 = Divide(x=w4, y=w14) -> (x/y=w3:dbl)
  "Total\nTemperature Change" <- w3
  n39 = Compound Arithmetic op=ADD(w133, w132, w130, w131, w129, w128, w22, w127, w126) -> (w169:dbl)
  "Mass 1 NS" <- w169
  n40 = Compound Arithmetic op=ADD(w143, w141, w139, w140, w138, w137, w136, w135, w134) -> (w172:dbl)
  "Volume 1 NS" <- w172
  n41 = Multiply(x=w169, y=2.0) -> (x*y=w168:dbl)
  "Mass 2 NS" <- w168
  n42 = Multiply(x=w172, y=2.0) -> (x*y=w171:dbl)
  "Vol 2 NS" <- w171
  n43 = Add(x=w168, y=w165) -> (x+y=w167:dbl)
  "Mass NS Pair with Gap" <- w167
  n44 = Add(x=w171, y=w166) -> (x+y=w170:dbl)
  "Volume NS Pair With Gap" <- w170
  n45 = Multiply(x=w170, y=w112) -> (x*y=w174:dbl)
  "Volume of a Chip" <- w174
  n46 = Multiply(x=w167, y=w112) -> (x*y=w173:dbl)
  "Mass of a Chip" <- w173
  n47 = call "EChem Signal.vi"("V_Zeta in"=w259, "Capacitance Functional Molecules per NS"=w213, "Series Resistance of Solution"=w31, "Frequency"=w30, "Freq Hz-MHz"=w29, "Capacitance Functional Analyte per NS"=w260, "C_EDL/ 1 NS"=w191) -> ("Impedance of EDL & Functionalization & Analyte"=w185:dbl, "Impedance of EDL & Functionalization"=w188:dbl, "Capacitance of ELD & Functionalization"=w187:dbl, "Total Impedance Rs+C(EDS+Funct)"=w184:dbl, "Capacitance of ELD & Functionalization & Analyte"=w186:dbl, "Total Impedance Rs+C(EDS+Funct+Analyte)"=w183:dbl, "Delta C"=w181:dbl, "Delta Total Impedance"=w182:dbl, "V_Zeta out"=w178:dbl, "Max i;  R+ C (EDL+Funct)"=w177:dbl, "|Z| of R+ C (EDL+Funct)"=w180:dbl, "Delta i"=w175:dbl, "Max i;  R+ C (EDL+Funct+ Analyte)"=w176:dbl, "|Z| of R+ C (EDL+Funct+Analyte)"=w179:dbl)  [unwired: 7 in]
  "Capacitance of ELD & Functionalization" <- w187
  "Capacitance of ELD & Functionalization & Analyte" <- w186
  "Delta C" <- w181
  "Impedance of EDL & Functionalization" <- w188
  "Impedance of EDL & Functionalization & Analyte" <- w185
  "Total Impedance Rs+C(EDS+Funct)" <- w184
  "Total Impedance Rs+C(EDS+Funct+Analyte)" <- w183
  "Delta Total Impedance" <- w182
  "|Z| of R+ C (EDL+Funct)" <- w180
  "|Z| of R+ C (EDL+Funct+Analyte)" <- w179
  "V_Zeta" <- w178
  "Max i;  R+ C (EDL+Funct)" <- w177
  "Max i;  R+ C (EDL+Funct+ Analyte)" <- w176
  "Delta i" <- w175
  n48 = Divide(x=w237, y=3600.0) -> (x/y=w236:dbl)
  "Chip Energy Wh" <- w236
  n49 = Divide(x=w237, y=w173) -> (x/y=w239:dbl)
  "Chip Energy /Mass" <- w239
  n50 = Divide(x=w237, y=w174) -> (x/y=w238:dbl)
  "Chip Energy / Volume" <- w238
  n51 = Divide(x=w244, y=w167) -> (x/y=w243:dbl)
  "1 NS Pair Energy / mass" <- w243
  n52 = Divide(x=w244, y=w170) -> (x/y=w242:dbl)
  "1 NS Pair Energy / Volume" <- w242
  n53 = Divide(x=w238, y=3600.0) -> (x/y=w234:dbl)
  "WH/m3" <- w234
  n54 = Divide(x=w239, y=3600.0) -> (x/y=w235:dbl)
  "WH/Kg" <- w235
  n55 = Divide(x=w234, y=1000.0) -> (x/y=w232:dbl)
  "WH/Lit" <- w232
  n56 = Divide(x=w32, y=w176) -> (x/y=w189:dbl)
  "Rf for Max i;  R+ C (EDL+Funct+ Analyte)" <- w189
  n57 = Divide(x=w32, y=w177) -> (x/y=w190:dbl)
  "Rf for Max i;  R+ C (EDL+Funct)" <- w190
  n58 = Multiply(x=w37, y=1000.0) -> (x*y=w231:dbl)
  "Energy Density  WH/m3" <- w231
  n59 = Multiply(x=w231, y=w170) -> (x*y=w229:dbl)
  "Energy (wh/m3) / 1 NS pari with gap" <- w229
  n60 = Multiply(x=3600.0, y=w229) -> (x*y=w230:dbl)
  "J in 1 NS pair with gap" <- w230
  n61 = Cast Unit Bases(0:w210, 1:w205) -> (2:w211:ext)
  n62 = To Double Precision Float(number=w211) -> (double precision float=w209:dbl)
  n63 = Cast Unit Bases(0:w207, 1:w205) -> (2:w208:ext)
  n64 = To Double Precision Float(number=w208) -> (double precision float=w206:dbl)
  n65 = Bundle("Capacitance of 1 Pair NS"=w245, "Energy"=w244, w243, w242, "Impedance"=w241, "Power"=w240, w239, w238, "Chip Capacitance"=w20, "Chip Energy"=w237, w236, w235, w234, "Chip Impedance"=w15, "Chip Power"=w233, w232, w231, w230, w229, "Volume of Molecule"=w228, "Area of Molecule on CNT surface"=w227, "Molecle Area with Gap"=w226, "Molecule Length"=w225, "Capacitance Functinal Analyte  per unit area"=w224, "Capaciatance per CNT"=w223, "Capacitance Functional Analyte per NS 2"=w222, "Capacitance Functional Analyte per NS 2"=w222, "Volume of Molecule"=w221, "Area of Molecule on CNT surface"=w220, "Molecle Area with Gap"=w219, "Molecule Length"=w218, "No of Molecules on 1 CNT Functionalized"=w217, "Total Functionalized Molecules on NS"=w216, w209, w206, "Capacitance Functinal Molecule  per unit area"=w215, "Capaciatance per CNT"=w214, "Capacitance Functional Molecules per NS"=w213, "Capacitance Functional Molecules per NS 2"=w212, "eo; Permitivity of Free Space"=w203, "c; Charge on e"=w202, "F=eN_a"=w201, "k; Boltzmann Constant"=w200, "N_a; Avagadro no"=w199, "R=kN_a"=w198, "C in M"=w197, "C_EDL/ A"=w196, "d; EDL Length"=w195, "C EDL by d"=w194, "C EDL by d with Cosh Factor"=w193, "C_EDL/ 1 CNT"=w192, "C_EDL/ 1 NS"=w191, w190, w189, "Capacitance of ELD & Functionalization"=w187, "Impedance of EDL & Functionalization"=w188, "Capacitance of ELD & Functionalization & Analyte"=w186, "Impedance of EDL & Functionalization & Analyte"=w185, "Total Impedance Rs+C(EDS+Funct)"=w184, "Total Impedance Rs+C(EDS+Funct+Analyte)"=w183, "Delta Total Impedance"=w182, "Delta C"=w181, "|Z| of R+ C (EDL+Funct)"=w180, "|Z| of R+ C (EDL+Funct+Analyte)"=w179, "V_Zeta out"=w178, "Max i;  R+ C (EDL+Funct)"=w177, "Max i;  R+ C (EDL+Funct+ Analyte)"=w176, "Delta i"=w175, w174, w173, w172, w171, w170, w169, w168, w167, w166, w165, "Silicon Thickness out"=w164, "Sio2 Thickness"=w163, "Dielectric Thickness  out"=w162, "Volume Si"=w161, "Volume SiO2"=w160, "Volume Dielectric"=w159, "Mass Si"=w158, "Mass SiO2"=w157, "Mass Dielectric"=w156, "Delta Temp Change Si"=w155, "Delta Temp Change SiO2"=w154, "Delta Temp Change \nDielectric"=w153, "Array Input[1]"=w81, w152, "Array Input[4]"=w78, "Array Input[29]"=w54, "Silicon Thickness out"=w151, "Sio2 Thickness"=w142, "SiO2 Thickness 2"=w150, "M1 Thickness"=w149, "Al2O3 Thickness"=w148, "Al Thickness"=w147, "Fe Thickness 2"=w146, "CNT Thickness"=w145, "Dielectric Thickness  out"=w144, "Volume Si"=w143, "Volume SiO2"=w141, "Volume SiO2 2"=w140, "Volume M1"=w139, "Volume Al2O3"=w138, "Volume Al"=w137, "Volume Fe"=w136, "Volume CNT"=w135, "Volume Dielectric"=w134, "Mass Si"=w133, "Mass SiO2"=w132, "Mass SiO2 2"=w131, "Mass M1"=w130, "Mass Al2O3"=w129, "Mass  Al"=w128, "Mass Fe"=w22, "Mass CNTs"=w127, "Mass Dielectric"=w126, "Delta Temp Change Si"=w125, "Delta Temp Change SiO2"=w124, "Delta Temp Change SiO2 2"=w123, "Delta Temp Change M1"=w122, "Delta Temp Change Al2O3"=w121, "Delta Temp Change Al"=w120, "Delta Temp Change Fe"=w119, "Delta Temp Change CNT"=w118, "Delta Temp Change \nDielectric"=w117, w4, "y"=w116, w115, w114, "Gap B/w NS"=w113, "No of NS Pairs on Chip"=w112, "NS Width"=w111, "NS Length"=w110, "NS Base Area"=w109, "Surface Area 1 NS"=w108, "# of CNTs in 1 NS"=w107, "Length of CNTs"=w106, "CNT Radius"=w105, "CNT Base Area"=w104, "Surface Area of 1 CNT"=w103, "Area 1 CNT & Gap"=w102, "Silicon Density"=w101, "SilO2 Density"=w100, "SilO2 Density 2"=w99, "M1 Density"=w98, "Al2O3 Density"=w97, "Al Density"=w96, "Fe Density"=w95, "CNT Density"=w94, "Dielectric Density"=w93, "Silicon Specfic Heat Capacity"=w92, "SiO2 Specfic Heat Capacity"=w91, "SiO2 Specfic Heat Capacity 2"=w90, "M1 Specfic Heat Capacity"=w89, "Al2O3 Specfic Heat Capacity"=w88, "Al Specfic Heat Capacity"=w87, "Fe Specfic Heat Capacity"=w86, "CNT Specfic Heat Capacity"=w85, "Dielectric Specfic Heat Capacity"=w84, w2, w1, w4, w3) -> (w83:T2)  [unwired: 1 in]
  n66 = Cluster To Array(cluster=w83) -> (array=→"Array Output":dbl[])
  "um in 1 inch" <- w116
